vi "Sleep Box.vi"() -> ()   [LabVIEW 2013]
uses:
  <vilib>/DAQmx/write.llb/DAQmx Write (Analog DBL 1Chan 1Samp).vi
  <vilib>/DAQmx/write.llb/DAQmx Write (Digital Bool 1Line 1Point).vi
  <vilib>/DAQmx/miscellaneous.llb/DAQmx Fill In Error Info.vi
panel:
  out "time log 2":refnum<file>
  out "time log":refnum<file>
  out "doQueue2":refnum<queue>
  out "doQueue1":refnum<queue>
  out "camera2":refnum<queue>
  out "camera1":refnum<queue>
  out "integral2":refnum<queue>
  out "integral1":refnum<queue>
  out "centroids2":refnum<queue>
  out "centroids1":refnum<queue>
  out "display2":refnum<queue>
  out "display1":refnum<queue>
  out "threshDisplay2":refnum<queue>
  out "threshDisplay1":refnum<queue>
  in  "roi data cluster 2":T1
  out "ROIs 2":T1={[0, 0, 1280, 960], [{"Contour Type"=0, "ROI Type"=12, [49, 61, 150, 162, 270516]}, {"Contour Type"=0, "ROI Type"=12, [50, 163, 151, 264, 270516]}, {"Contour Type"=0, "ROI Type"=12, [51, 264, 152, 365, 270516]}, {"Contour Type"=0, "ROI Type"=12, [52, 366, 153, 467, 270516]}, {"Contour Type"=0, "ROI Type"=12, [52, 468, 154, 568, 270516]}, {"Contour Type"=0, "ROI Type"=12, [53, 569, 154, 670, 270516]}, {"Contour Type"=0, "ROI Type"=12, [54, 671, 155, 772, 270516]}, {"Contour Type"=0, "ROI Type"=12, [55, 772, 156, 873, 270516]}, {"Contour Type"=0, "ROI Type"=12, [151, 60, 252, 161, 270516]}, {"Contour Type"=0, "ROI Type"=12, [152, 162, 253, 263, 270516]}, {"Contour Type"=0, "ROI Type"=12, [153, 263, 254, 364, 270516]}, {"Contour Type"=0, "ROI Type"=12, [153, 365, 254, 466, 270516]}, {"Contour Type"=0, "ROI Type"=12, [154, 467, 255, 568, 270516]}, {"Contour Type"=0, "ROI Type"=12, [155, 568, 256, 669, 270516]}, {"Contour Type"=0, "ROI Type"=12, [156, 670, 257, 771, 270516]}, {"Contour Type"=0, "ROI Type"=12, [157, 771, 258, 872, 270516]}, {"Contour Type"=0, "ROI Type"=12, [253, 59, 354, 160, 270516]}, {"Contour Type"=0, "ROI Type"=12, [254, 161, 355, 262, 270516]}, {"Contour Type"=0, "ROI Type"=12, [254, 262, 355, 363, 270516]}, {"Contour Type"=0, "ROI Type"=12, [255, 364, 356, 465, 270516]}, {"Contour Type"=0, "ROI Type"=12, [256, 466, 357, 567, 270516]}, {"Contour Type"=0, "ROI Type"=12, [257, 567, 358, 668, 270516]}, {"Contour Type"=0, "ROI Type"=12, [258, 669, 359, 770, 270516]}, {"Contour Type"=0, "ROI Type"=12, [259, 771, 360, 872, 270516]}, {"Contour Type"=0, "ROI Type"=12, [354, 58, 456, 159, 270516]}, {"Contour Type"=0, "ROI Type"=12, [355, 160, 456, 261, 270516]}, {"Contour Type"=0, "ROI Type"=12, [356, 262, 457, 362, 270516]}, {"Contour Type"=0, "ROI Type"=12, [357, 363, 458, 464, 270516]}, {"Contour Type"=0, "ROI Type"=12, [358, 465, 459, 566, 270516]}, {"Contour Type"=0, "ROI Type"=12, [359, 566, 460, 667, 270516]}, {"Contour Type"=0, "ROI Type"=12, [360, 668, 461, 769, 270516]}, {"Contour Type"=0, "ROI Type"=12, [361, 770, 462, 871, 270516]}, {"Contour Type"=0, "ROI Type"=12, [456, 57, 557, 158, 270516]}, {"Contour Type"=0, "ROI Type"=12, [457, 159, 558, 260, 270516]}, {"Contour Type"=0, "ROI Type"=12, [458, 261, 559, 362, 270516]}, {"Contour Type"=0, "ROI Type"=12, [459, 362, 560, 463, 270516]}, {"Contour Type"=0, "ROI Type"=12, [460, 464, 561, 565, 270516]}, {"Contour Type"=0, "ROI Type"=12, [461, 565, 562, 666, 270516]}, {"Contour Type"=0, "ROI Type"=12, [462, 667, 563, 768, 270516]}, {"Contour Type"=0, "ROI Type"=12, [462, 769, 563, 870, 270516]}, {"Contour Type"=0, "ROI Type"=12, [558, 56, 659, 157, 270516]}, {"Contour Type"=0, "ROI Type"=12, [559, 158, 660, 259, 270516]}, {"Contour Type"=0, "ROI Type"=12, [560, 260, 661, 361, 270516]}, {"Contour Type"=0, "ROI Type"=12, [561, 361, 662, 462, 270516]}, {"Contour Type"=0, "ROI Type"=12, [562, 463, 663, 564, 270516]}, {"Contour Type"=0, "ROI Type"=12, [563, 565, 664, 666, 270516]}, {"Contour Type"=0, "ROI Type"=12, [563, 666, 664, 767, 270516]}, {"Contour Type"=0, "ROI Type"=12, [564, 768, 665, 869, 270516]}, {"Contour Type"=0, "ROI Type"=12, [660, 56, 761, 156, 270516]}, {"Contour Type"=0, "ROI Type"=12, [661, 157, 762, 258, 270516]}, {"Contour Type"=0, "ROI Type"=12, [662, 259, 763, 360, 270516]}, {"Contour Type"=0, "ROI Type"=12, [663, 360, 764, 461, 270516]}, {"Contour Type"=0, "ROI Type"=12, [664, 462, 764, 563, 270516]}, {"Contour Type"=0, "ROI Type"=12, [664, 564, 765, 665, 270516]}, {"Contour Type"=0, "ROI Type"=12, [665, 665, 766, 766, 270516]}, {"Contour Type"=0, "ROI Type"=12, [666, 767, 767, 868, 270516]}, {"Contour Type"=0, "ROI Type"=12, [762, 55, 863, 156, 270516]}, {"Contour Type"=0, "ROI Type"=12, [763, 156, 864, 257, 270516]}, {"Contour Type"=0, "ROI Type"=12, [764, 258, 865, 359, 270516]}, {"Contour Type"=0, "ROI Type"=12, [764, 359, 865, 460, 270516]}, {"Contour Type"=0, "ROI Type"=12, [765, 461, 866, 562, 270516]}, {"Contour Type"=0, "ROI Type"=12, [766, 563, 867, 664, 270516]}, {"Contour Type"=0, "ROI Type"=12, [767, 664, 868, 765, 270516]}, {"Contour Type"=0, "ROI Type"=12, [768, 766, 869, 867, 270516]}, {"Contour Type"=0, "ROI Type"=12, [864, 54, 965, 155, 270516]}, {"Contour Type"=0, "ROI Type"=12, [865, 155, 966, 256, 270516]}, {"Contour Type"=0, "ROI Type"=12, [865, 257, 966, 358, 270516]}, {"Contour Type"=0, "ROI Type"=12, [866, 359, 967, 460, 270516]}, {"Contour Type"=0, "ROI Type"=12, [867, 460, 968, 561, 270516]}, {"Contour Type"=0, "ROI Type"=12, [868, 562, 969, 663, 270516]}, {"Contour Type"=0, "ROI Type"=12, [869, 663, 970, 764, 270516]}, {"Contour Type"=0, "ROI Type"=12, [870, 765, 971, 866, 270516]}, {"Contour Type"=0, "ROI Type"=12, [966, 53, 1066, 154, 270516]}, {"Contour Type"=0, "ROI Type"=12, [966, 154, 1067, 255, 270516]}, {"Contour Type"=0, "ROI Type"=12, [967, 256, 1068, 357, 270516]}, {"Contour Type"=0, "ROI Type"=12, [968, 358, 1069, 459, 270516]}, {"Contour Type"=0, "ROI Type"=12, [969, 459, 1070, 560, 270516]}, {"Contour Type"=0, "ROI Type"=12, [970, 561, 1071, 662, 270516]}, {"Contour Type"=0, "ROI Type"=12, [971, 662, 1072, 764, 270516]}, {"Contour Type"=0, "ROI Type"=12, [972, 764, 1073, 865, 270516]}, {"Contour Type"=0, "ROI Type"=12, [1067, 52, 1168, 153, 270516]}, {"Contour Type"=0, "ROI Type"=12, [1068, 153, 1169, 254, 270516]}, {"Contour Type"=0, "ROI Type"=12, [1069, 255, 1170, 356, 270516]}, {"Contour Type"=0, "ROI Type"=12, [1070, 357, 1171, 458, 270516]}, {"Contour Type"=0, "ROI Type"=12, [1071, 458, 1172, 559, 270516]}, {"Contour Type"=0, "ROI Type"=12, [1072, 560, 1173, 661, 270516]}, {"Contour Type"=0, "ROI Type"=12, [1073, 662, 1174, 763, 270516]}, {"Contour Type"=0, "ROI Type"=12, [1073, 763, 1174, 864, 270516]}, {"Contour Type"=0, "ROI Type"=12, [1169, 51, 1270, 152, 270516]}, {"Contour Type"=0, "ROI Type"=12, [1170, 153, 1271, 254, 270516]}, {"Contour Type"=0, "ROI Type"=12, [1171, 254, 1272, 355, 270516]}, {"Contour Type"=0, "ROI Type"=12, [1172, 356, 1273, 457, 270516]}, {"Contour Type"=0, "ROI Type"=12, [1173, 457, 1274, 558, 270516]}, {"Contour Type"=0, "ROI Type"=12, [1174, 559, 1275, 660, 270516]}, {"Contour Type"=0, "ROI Type"=12, [1174, 661, 1275, 762, 270516]}, {"Contour Type"=0, "ROI Type"=12, [1175, 762, 1276, 863, 270516]}]}
  out "centroid log 2":refnum<file>
  out "motion log 2":refnum<file>
  in  "Tab Control":enum32{"Main View", "Files to load/save"}(tab)=enum."Files to load/save"
  out "Image":T2(plugin-control)
  in  "Camera":bool=TRUE
  in  "Ring":u16(ring) items=["Raw", "Diff Threshold", "Integrated Motion"]
  in  "stop":bool
  out "Buffers":i32(slide) scale=0.0..100.0
  out "Intensity Graph":u32[][](graph)
  out "frame#1":i32
  out "frame#2":i32
  in  "ROI Refernce Image 2":path=path "C:/Users/SleepBox/Desktop/072516_Box4.bmp"
  in  "ROI Refernce Image 1":path=path "C:/Users/SleepBox/Desktop/072516_Box3.bmp"
  in  "Load Experimental Parameters 2":path=path "C:/Users/SleepBox/Desktop/072516_TapsFlashes_Box4_Complete.csv"
  in  "Load ROI Data 2":path=path "C:/Users/SleepBox/Desktop/072516_Box4_ROI"
  in  "Log File Base Name 2":path=path "C:/Users/SleepBox/Desktop/testlog"
  in  "Load Experimental Parameters":path=path "C:/Users/SleepBox/Desktop/072516_TapsFlashes_Box3_Complete.csv"
  in  "Load ROI Data":path=path "C:/Users/SleepBox/Desktop/072516_Box3_ROI"
  in  "Log File Base Name":path=path "C:/Users/SleepBox/Desktop/testlog"
  in  "diff threshold":dbl=3.0
  out "event log":refnum<file>
  out "event log 2":refnum<file>
  out "motion log":refnum<file>
  out "centroid log":refnum<file>
  out "ROIs":T1={[0, 0, 1280, 960], [{"Contour Type"=0, "ROI Type"=12, [49, 61, 150, 162, 270516]}, {"Contour Type"=0, "ROI Type"=12, [50, 163, 151, 264, 270516]}, {"Contour Type"=0, "ROI Type"=12, [51, 264, 152, 365, 270516]}, {"Contour Type"=0, "ROI Type"=12, [52, 366, 153, 467, 270516]}, {"Contour Type"=0, "ROI Type"=12, [52, 468, 154, 568, 270516]}, {"Contour Type"=0, "ROI Type"=12, [53, 569, 154, 670, 270516]}, {"Contour Type"=0, "ROI Type"=12, [54, 671, 155, 772, 270516]}, {"Contour Type"=0, "ROI Type"=12, [55, 772, 156, 873, 270516]}, {"Contour Type"=0, "ROI Type"=12, [151, 60, 252, 161, 270516]}, {"Contour Type"=0, "ROI Type"=12, [152, 162, 253, 263, 270516]}, {"Contour Type"=0, "ROI Type"=12, [153, 263, 254, 364, 270516]}, {"Contour Type"=0, "ROI Type"=12, [153, 365, 254, 466, 270516]}, {"Contour Type"=0, "ROI Type"=12, [154, 467, 255, 568, 270516]}, {"Contour Type"=0, "ROI Type"=12, [155, 568, 256, 669, 270516]}, {"Contour Type"=0, "ROI Type"=12, [156, 670, 257, 771, 270516]}, {"Contour Type"=0, "ROI Type"=12, [157, 771, 258, 872, 270516]}, {"Contour Type"=0, "ROI Type"=12, [253, 59, 354, 160, 270516]}, {"Contour Type"=0, "ROI Type"=12, [254, 161, 355, 262, 270516]}, {"Contour Type"=0, "ROI Type"=12, [254, 262, 355, 363, 270516]}, {"Contour Type"=0, "ROI Type"=12, [255, 364, 356, 465, 270516]}, {"Contour Type"=0, "ROI Type"=12, [256, 466, 357, 567, 270516]}, {"Contour Type"=0, "ROI Type"=12, [257, 567, 358, 668, 270516]}, {"Contour Type"=0, "ROI Type"=12, [258, 669, 359, 770, 270516]}, {"Contour Type"=0, "ROI Type"=12, [259, 771, 360, 872, 270516]}, {"Contour Type"=0, "ROI Type"=12, [354, 58, 456, 159, 270516]}, {"Contour Type"=0, "ROI Type"=12, [355, 160, 456, 261, 270516]}, {"Contour Type"=0, "ROI Type"=12, [356, 262, 457, 362, 270516]}, {"Contour Type"=0, "ROI Type"=12, [357, 363, 458, 464, 270516]}, {"Contour Type"=0, "ROI Type"=12, [358, 465, 459, 566, 270516]}, {"Contour Type"=0, "ROI Type"=12, [359, 566, 460, 667, 270516]}, {"Contour Type"=0, "ROI Type"=12, [360, 668, 461, 769, 270516]}, {"Contour Type"=0, "ROI Type"=12, [361, 770, 462, 871, 270516]}, {"Contour Type"=0, "ROI Type"=12, [456, 57, 557, 158, 270516]}, {"Contour Type"=0, "ROI Type"=12, [457, 159, 558, 260, 270516]}, {"Contour Type"=0, "ROI Type"=12, [458, 261, 559, 362, 270516]}, {"Contour Type"=0, "ROI Type"=12, [459, 362, 560, 463, 270516]}, {"Contour Type"=0, "ROI Type"=12, [460, 464, 561, 565, 270516]}, {"Contour Type"=0, "ROI Type"=12, [461, 565, 562, 666, 270516]}, {"Contour Type"=0, "ROI Type"=12, [462, 667, 563, 768, 270516]}, {"Contour Type"=0, "ROI Type"=12, [462, 769, 563, 870, 270516]}, {"Contour Type"=0, "ROI Type"=12, [558, 56, 659, 157, 270516]}, {"Contour Type"=0, "ROI Type"=12, [559, 158, 660, 259, 270516]}, {"Contour Type"=0, "ROI Type"=12, [560, 260, 661, 361, 270516]}, {"Contour Type"=0, "ROI Type"=12, [561, 361, 662, 462, 270516]}, {"Contour Type"=0, "ROI Type"=12, [562, 463, 663, 564, 270516]}, {"Contour Type"=0, "ROI Type"=12, [563, 565, 664, 666, 270516]}, {"Contour Type"=0, "ROI Type"=12, [563, 666, 664, 767, 270516]}, {"Contour Type"=0, "ROI Type"=12, [564, 768, 665, 869, 270516]}, {"Contour Type"=0, "ROI Type"=12, [660, 56, 761, 156, 270516]}, {"Contour Type"=0, "ROI Type"=12, [661, 157, 762, 258, 270516]}, {"Contour Type"=0, "ROI Type"=12, [662, 259, 763, 360, 270516]}, {"Contour Type"=0, "ROI Type"=12, [663, 360, 764, 461, 270516]}, {"Contour Type"=0, "ROI Type"=12, [664, 462, 764, 563, 270516]}, {"Contour Type"=0, "ROI Type"=12, [664, 564, 765, 665, 270516]}, {"Contour Type"=0, "ROI Type"=12, [665, 665, 766, 766, 270516]}, {"Contour Type"=0, "ROI Type"=12, [666, 767, 767, 868, 270516]}, {"Contour Type"=0, "ROI Type"=12, [762, 55, 863, 156, 270516]}, {"Contour Type"=0, "ROI Type"=12, [763, 156, 864, 257, 270516]}, {"Contour Type"=0, "ROI Type"=12, [764, 258, 865, 359, 270516]}, {"Contour Type"=0, "ROI Type"=12, [764, 359, 865, 460, 270516]}, {"Contour Type"=0, "ROI Type"=12, [765, 461, 866, 562, 270516]}, {"Contour Type"=0, "ROI Type"=12, [766, 563, 867, 664, 270516]}, {"Contour Type"=0, "ROI Type"=12, [767, 664, 868, 765, 270516]}, {"Contour Type"=0, "ROI Type"=12, [768, 766, 869, 867, 270516]}, {"Contour Type"=0, "ROI Type"=12, [864, 54, 965, 155, 270516]}, {"Contour Type"=0, "ROI Type"=12, [865, 155, 966, 256, 270516]}, {"Contour Type"=0, "ROI Type"=12, [865, 257, 966, 358, 270516]}, {"Contour Type"=0, "ROI Type"=12, [866, 359, 967, 460, 270516]}, {"Contour Type"=0, "ROI Type"=12, [867, 460, 968, 561, 270516]}, {"Contour Type"=0, "ROI Type"=12, [868, 562, 969, 663, 270516]}, {"Contour Type"=0, "ROI Type"=12, [869, 663, 970, 764, 270516]}, {"Contour Type"=0, "ROI Type"=12, [870, 765, 971, 866, 270516]}, {"Contour Type"=0, "ROI Type"=12, [966, 53, 1066, 154, 270516]}, {"Contour Type"=0, "ROI Type"=12, [966, 154, 1067, 255, 270516]}, {"Contour Type"=0, "ROI Type"=12, [967, 256, 1068, 357, 270516]}, {"Contour Type"=0, "ROI Type"=12, [968, 358, 1069, 459, 270516]}, {"Contour Type"=0, "ROI Type"=12, [969, 459, 1070, 560, 270516]}, {"Contour Type"=0, "ROI Type"=12, [970, 561, 1071, 662, 270516]}, {"Contour Type"=0, "ROI Type"=12, [971, 662, 1072, 764, 270516]}, {"Contour Type"=0, "ROI Type"=12, [972, 764, 1073, 865, 270516]}, {"Contour Type"=0, "ROI Type"=12, [1067, 52, 1168, 153, 270516]}, {"Contour Type"=0, "ROI Type"=12, [1068, 153, 1169, 254, 270516]}, {"Contour Type"=0, "ROI Type"=12, [1069, 255, 1170, 356, 270516]}, {"Contour Type"=0, "ROI Type"=12, [1070, 357, 1171, 458, 270516]}, {"Contour Type"=0, "ROI Type"=12, [1071, 458, 1172, 559, 270516]}, {"Contour Type"=0, "ROI Type"=12, [1072, 560, 1173, 661, 270516]}, {"Contour Type"=0, "ROI Type"=12, [1073, 662, 1174, 763, 270516]}, {"Contour Type"=0, "ROI Type"=12, [1073, 763, 1174, 864, 270516]}, {"Contour Type"=0, "ROI Type"=12, [1169, 51, 1270, 152, 270516]}, {"Contour Type"=0, "ROI Type"=12, [1170, 153, 1271, 254, 270516]}, {"Contour Type"=0, "ROI Type"=12, [1171, 254, 1272, 355, 270516]}, {"Contour Type"=0, "ROI Type"=12, [1172, 356, 1273, 457, 270516]}, {"Contour Type"=0, "ROI Type"=12, [1173, 457, 1274, 558, 270516]}, {"Contour Type"=0, "ROI Type"=12, [1174, 559, 1275, 660, 270516]}, {"Contour Type"=0, "ROI Type"=12, [1174, 661, 1275, 762, 270516]}, {"Contour Type"=0, "ROI Type"=12, [1175, 762, 1276, 863, 270516]}]}
  in  "roi data cluster":T1
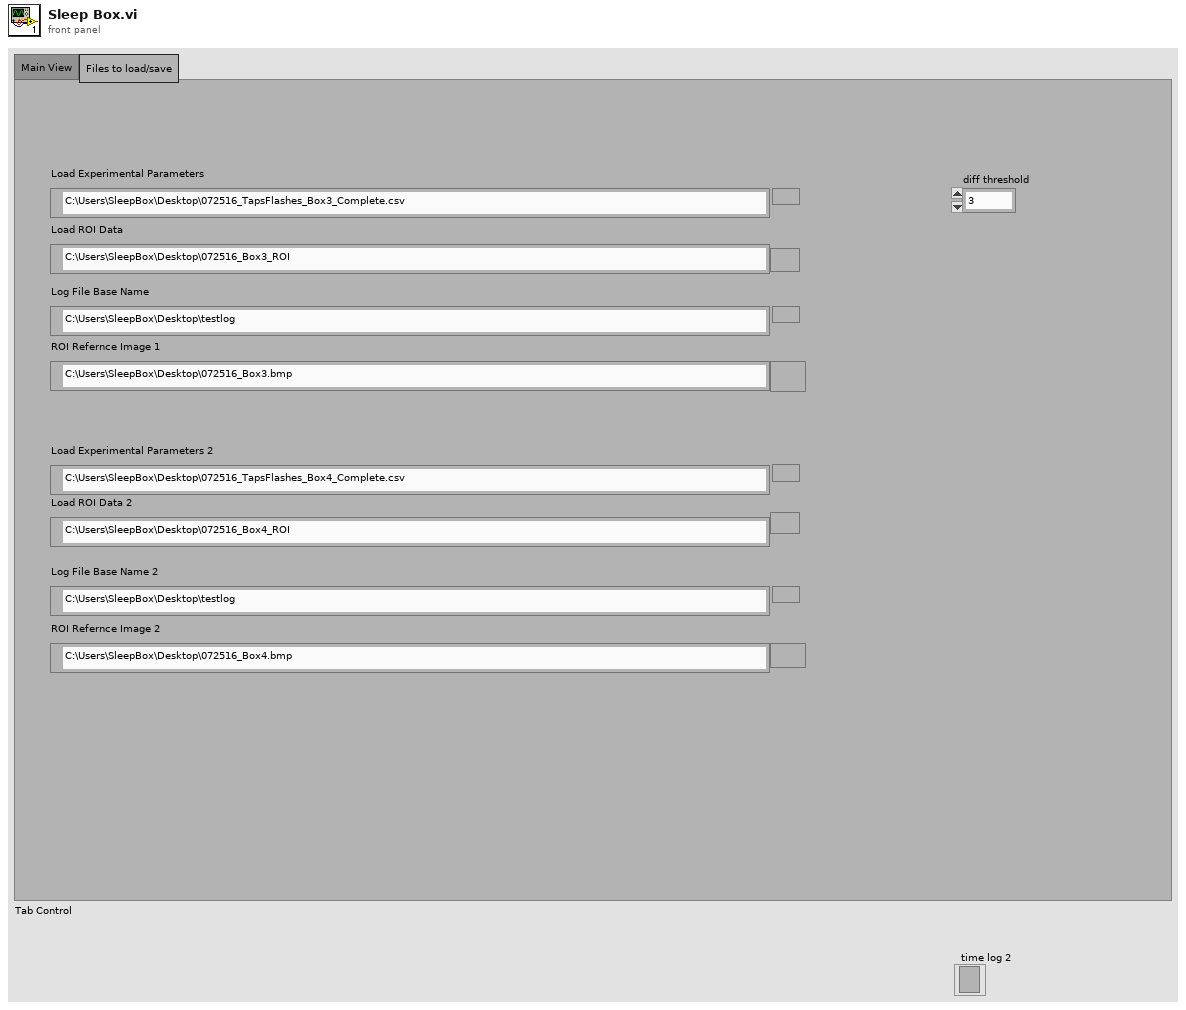
[diagram p1: front panel]
types:
  T1 = cluster{i32[], cluster{"Contour Type":u32, "ROI Type":u32, i32[]}[]}
  T2 = typedef "IMAQ Image.ctl" = refnum<image>
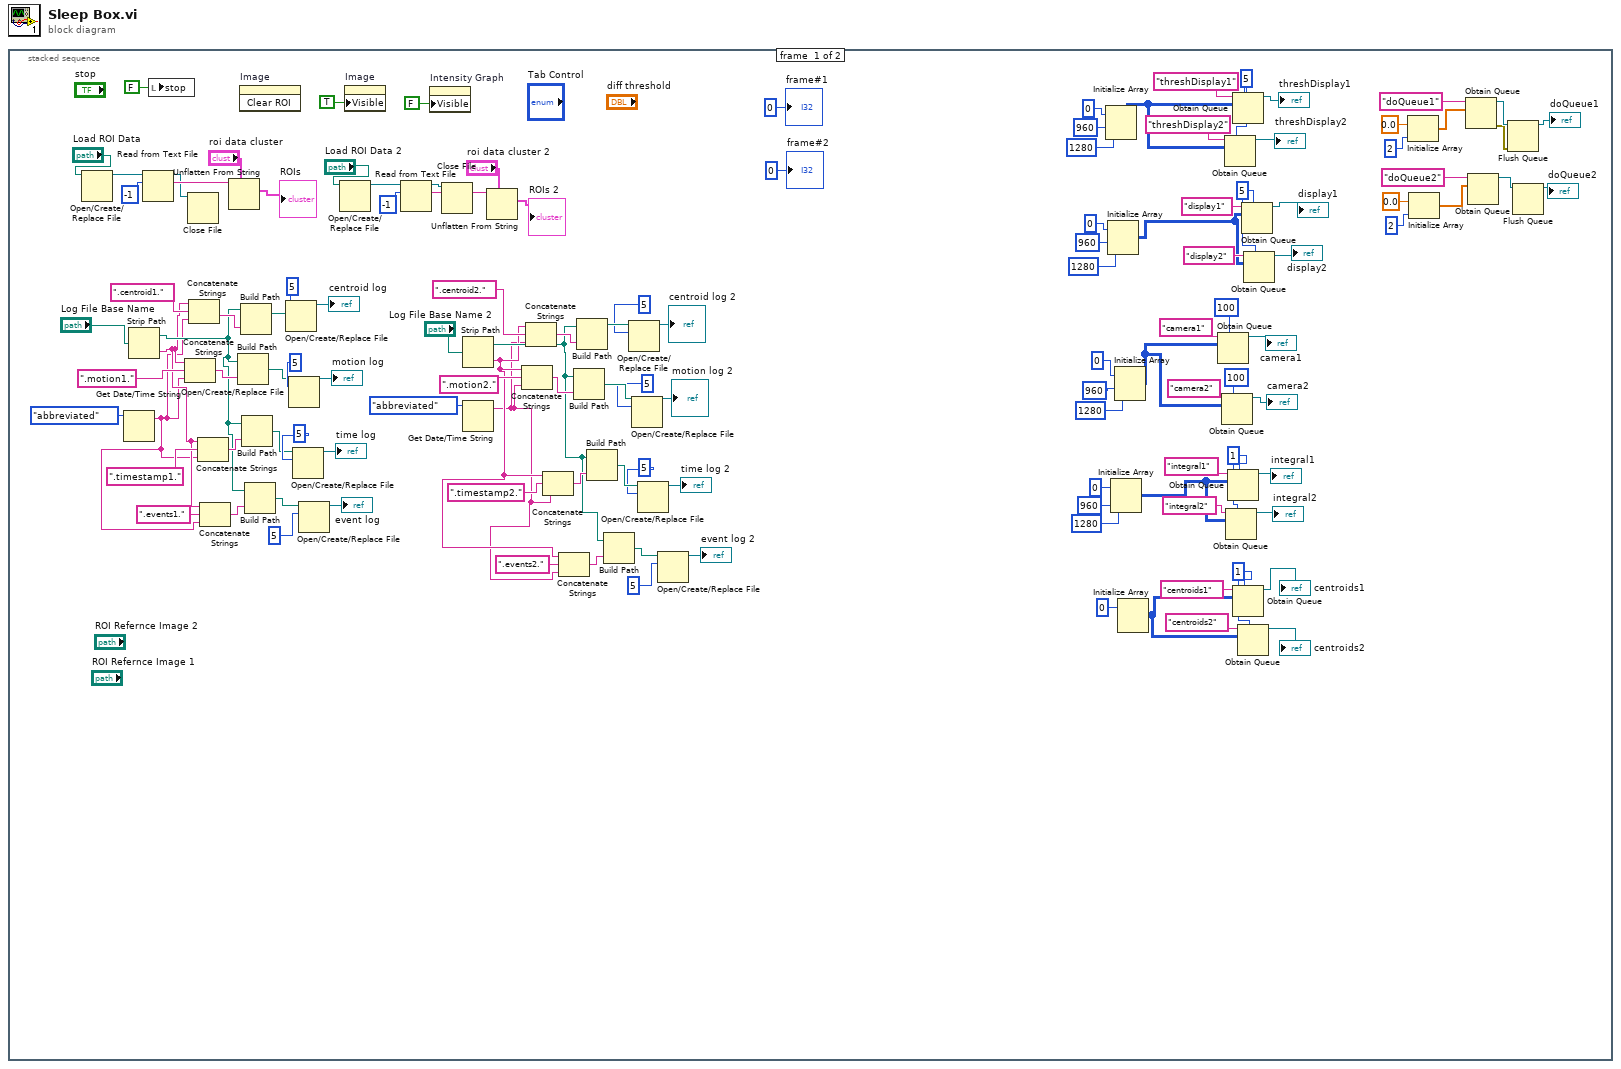
[diagram p0: block diagram]
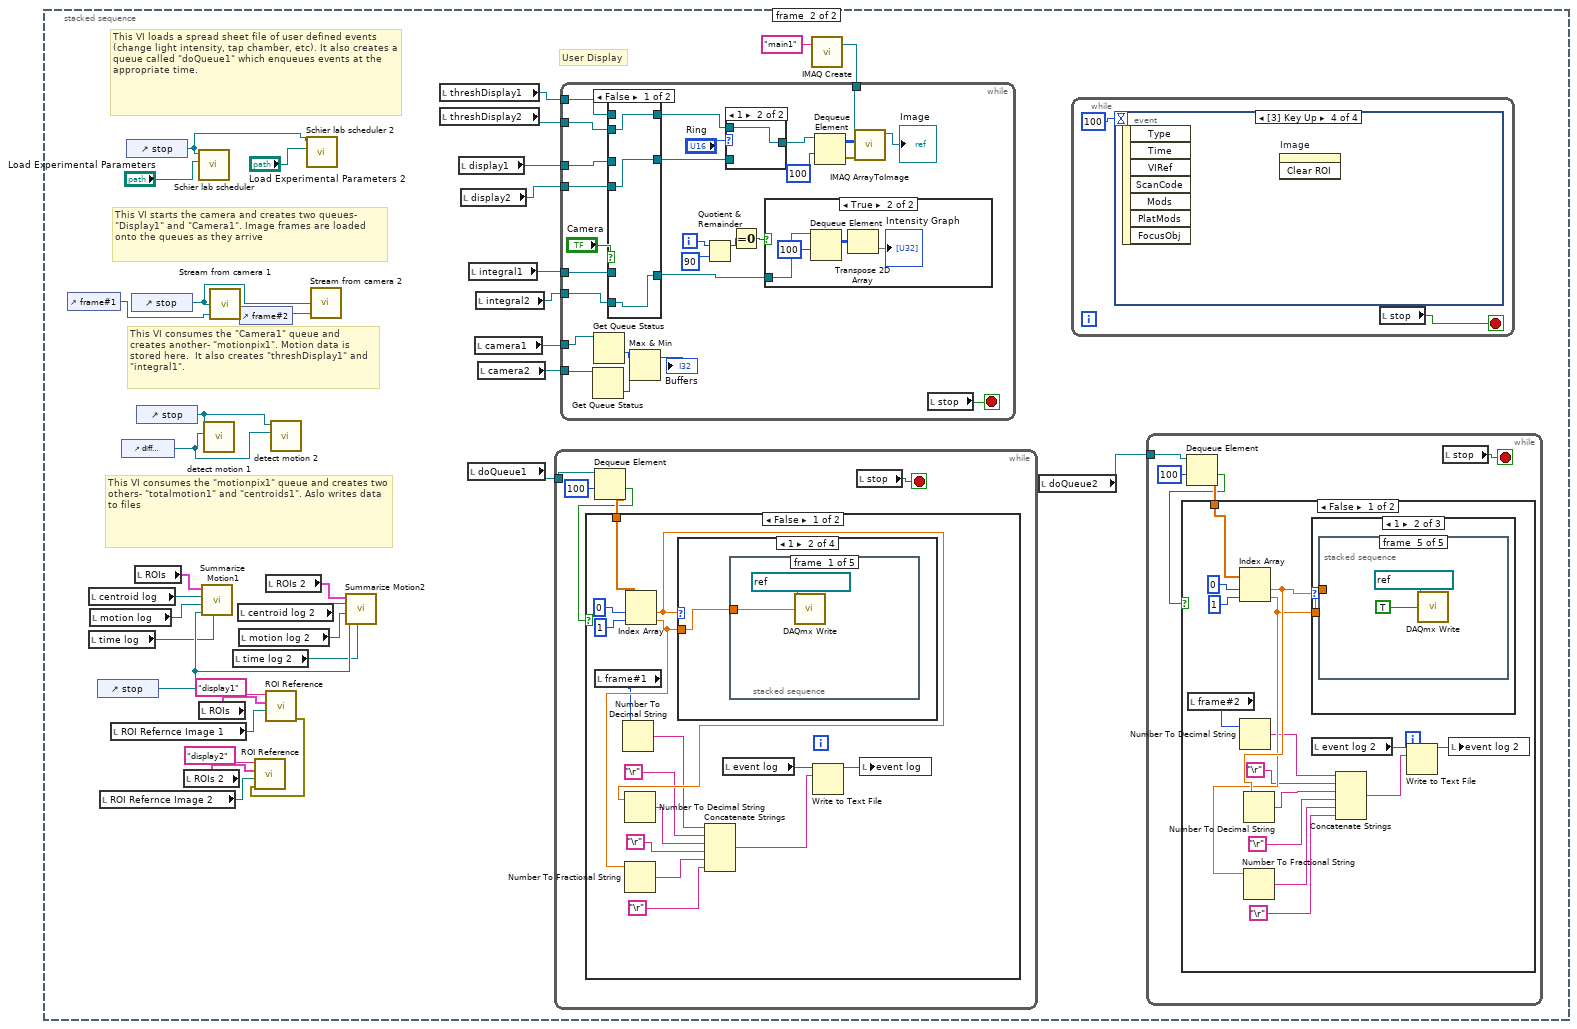
[diagram p2: hidden frame]
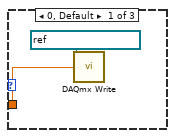
[diagram p3: hidden frame]
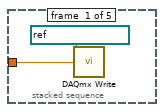
[diagram p4: hidden frame]
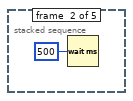
[diagram p5: hidden frame]
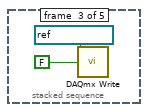
[diagram p6: hidden frame]
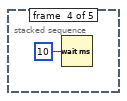
[diagram p7: hidden frame]
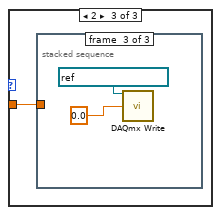
[diagram p8: hidden frame]
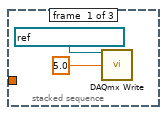
[diagram p9: hidden frame]
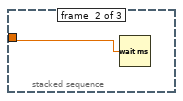
[diagram p10: hidden frame]
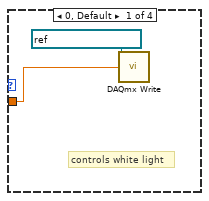
[diagram p12: hidden frame]
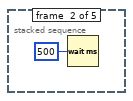
[diagram p13: hidden frame]
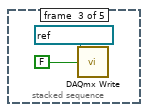
[diagram p14: hidden frame]
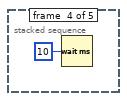
[diagram p15: hidden frame]
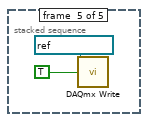
[diagram p16: hidden frame]
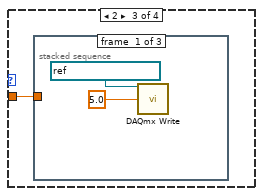
[diagram p17: hidden frame]
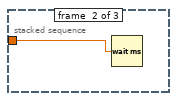
[diagram p18: hidden frame]
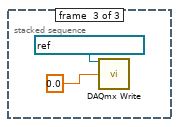
[diagram p19: hidden frame]
diagram:
  n1 = stacked-sequence {
    frame #0 {
      w46 = 1 ("max queue size (-1, unlimited)")
      w61 = 1 ("max queue size (-1, unlimited)")
      w70 = 5 ("max queue size (-1, unlimited)")
      w77 = 5 ("max queue size (-1, unlimited)")
      n2 = Open/Create/Replace File(file path (use dialog)="Load ROI Data") -> (refnum out=w121:refnum<file>)  [unwired: 5 in, 2 out]
      n3 = Get Date/Time String(date format (0)=enum16{"short", "long", "abbreviated"}."abbreviated") -> (date string=w18:string)  [unwired: 2 in, 1 out]
      n4 = Strip Path(path="Log File Base Name") -> (stripped path=w21:path, name=w20:string)
      n5 = Read from Text File(file (use dialog)=w121, count=-1) -> (refnum out=w123:refnum<file>, text=w124:string)  [unwired: 2 in, 2 out]
      n6 = local write "stop"(FALSE ("stop")) -> ()
      n7 = Concatenate Strings(w20, ".motion1.", w18) -> (w112:string)
      n8 = Close File(refnum=w123) -> ()  [unwired: 1 in, 2 out]
      n9 = Concatenate Strings(w20, ".centroid1.", w18) -> (w113:string)
      n10 = Concatenate Strings(w20, ".timestamp1." ("string"), w18) -> (w32:string)
      n11 = Concatenate Strings(w20, ".events1." ("string"), w18) -> (w23:string)
      n12 = Unflatten From String(type="roi data cluster", binary string=w124) -> (value=→"ROIs":T1)  [unwired: 3 in, 2 out]
      n13 = Build Path(base path=w21, name or relative path=w112) -> (appended path=w108:path)
      n14 = invoke on="Image" class="ImageControl" method="Clear ROI"() -> ()  [unwired: 3 in, 3 out]
      n15 = Build Path(base path=w21, name or relative path=w113) -> (appended path=w111:path)
      n16 = Build Path(base path=w21, name or relative path=w32) -> (appended path=w30:path)
      n17 = Build Path(base path=w21, name or relative path=w23) -> (appended path=w22:path)
      n18 = Open/Create/Replace File(file path (use dialog)=w111, operation (0:open)=5 ("count")) -> (refnum out=→"centroid log":refnum<file>)  [unwired: 4 in, 2 out]
      n19 = Open/Create/Replace File(file path (use dialog)=w108, operation (0:open)=5 ("count")) -> (refnum out=→"motion log":refnum<file>)  [unwired: 4 in, 2 out]
      n20 = Open/Create/Replace File(file path (use dialog)=w30, operation (0:open)=5 ("count")) -> (refnum out=→"time log":refnum<file>)  [unwired: 4 in, 2 out]
      n21 = Open/Create/Replace File(file path (use dialog)=w22, operation (0:open)=5 ("count")) -> (refnum out=→"event log":refnum<file>)  [unwired: 4 in, 2 out]
      n22 = Open/Create/Replace File(file path (use dialog)="Load ROI Data 2") -> (refnum out=w94:refnum<file>)  [unwired: 5 in, 2 out]
      n23 = property on="Image" class="ImageControl"("Visible"=TRUE) -> ()  [unwired: 2 in, 2 out]
      n24 = Read from Text File(file (use dialog)=w94, count=-1) -> (refnum out=w92:refnum<file>, text=w91:string)  [unwired: 2 in, 2 out]
      n25 = property on="Intensity Graph" class="IntGraph (strict)"("Visible"=FALSE) -> ()  [unwired: 2 in, 2 out]
      n26 = Close File(refnum=w92) -> ()  [unwired: 1 in, 2 out]
      n27 = Strip Path(path="Log File Base Name 2") -> (stripped path=w12:path, name=w11:string)
      n28 = Get Date/Time String(date format (0)=enum16{"short", "long", "abbreviated"}."abbreviated") -> (date string=w10:string)  [unwired: 2 in, 1 out]
      n29 = Unflatten From String(type="roi data cluster 2", binary string=w91) -> (value=→"ROIs 2":T1)  [unwired: 3 in, 2 out]
      n30 = Concatenate Strings(w11, ".motion2.", w10) -> (w103:string)
      n31 = Concatenate Strings(w11, ".centroid2.", w10) -> (w102:string)
      n32 = Concatenate Strings(w11, ".timestamp2." ("string"), w10) -> (w25:string)
      n33 = Concatenate Strings(w11, ".events2." ("string"), w10) -> (w13:string)
      n34 = Build Path(base path=w12, name or relative path=w103) -> (appended path=w107:path)
      n35 = Build Path(base path=w12, name or relative path=w102) -> (appended path=w104:path)
      n36 = Build Path(base path=w12, name or relative path=w25) -> (appended path=w27:path)
      n37 = Build Path(base path=w12, name or relative path=w13) -> (appended path=w14:path)
      n38 = Open/Create/Replace File(file path (use dialog)=w104, operation (0:open)=5 ("count")) -> (refnum out=→"centroid log 2":refnum<file>)  [unwired: 4 in, 2 out]
      n39 = Open/Create/Replace File(file path (use dialog)=w107, operation (0:open)=5 ("count")) -> (refnum out=→"motion log 2":refnum<file>)  [unwired: 4 in, 2 out]
      n40 = Open/Create/Replace File(file path (use dialog)=w27, operation (0:open)=5 ("count")) -> (refnum out=→"time log 2":refnum<file>)  [unwired: 4 in, 2 out]
      n41 = Open/Create/Replace File(file path (use dialog)=w14, operation (0:open)=5 ("count")) -> (refnum out=→"event log 2":refnum<file>)  [unwired: 4 in, 2 out]
      n42 = Initialize Array(u8 0 ("element"), 960 ("dimension size"), 1280 ("dimension size")) -> (w79:u8[][])
      n43 = Initialize Array(u8 0 ("element"), 960 ("dimension size"), 1280 ("dimension size")) -> (w69:u8[][])
      n44 = Initialize Array(u32 0 ("element"), 960 ("dimension size"), 1280 ("dimension size")) -> (w62:u32[][])
      n45 = Initialize Array(i16 0 ("element"), 960 ("dimension size"), 1280 ("dimension size")) -> (w42:i16[][])
      n46 = Initialize Array(u16 0 ("element")) -> (w45:u16[][])  [unwired: 2 in]
      n47 = Obtain Queue(max queue size (-1, unlimited)=100, name (unnamed)="camera1", element data type=w42) -> (queue out=→"camera1":refnum<queue>)  [unwired: 2 in, 2 out]
      n48 = Obtain Queue(max queue size (-1, unlimited)=100, name (unnamed)="camera2", element data type=w42) -> (queue out=→"camera2":refnum<queue>)  [unwired: 2 in, 2 out]
      n49 = Obtain Queue(max queue size (-1, unlimited)=w77, name (unnamed)="threshDisplay2", element data type=w79) -> (queue out=→"threshDisplay2":refnum<queue>)  [unwired: 2 in, 2 out]
      n50 = Obtain Queue(max queue size (-1, unlimited)=w61, name (unnamed)="integral2", element data type=w62) -> (queue out=→"integral2":refnum<queue>)  [unwired: 2 in, 2 out]
      n51 = Obtain Queue(max queue size (-1, unlimited)=w61, name (unnamed)="integral1", element data type=w62) -> (queue out=→"integral1":refnum<queue>)  [unwired: 2 in, 2 out]
      n52 = Obtain Queue(max queue size (-1, unlimited)=w77, name (unnamed)="threshDisplay1", element data type=w79) -> (queue out=→"threshDisplay1":refnum<queue>)  [unwired: 2 in, 2 out]
      n53 = Obtain Queue(max queue size (-1, unlimited)=w46, name (unnamed)="centroids1", element data type=w45) -> (queue out=→"centroids1":refnum<queue>)  [unwired: 2 in, 2 out]
      n54 = Obtain Queue(max queue size (-1, unlimited)=w46, name (unnamed)="centroids2", element data type=w45) -> (queue out=→"centroids2":refnum<queue>)  [unwired: 2 in, 2 out]
      n55 = Obtain Queue(max queue size (-1, unlimited)=w70, name (unnamed)="display1", element data type=w69) -> (queue out=→"display1":refnum<queue>)  [unwired: 2 in, 2 out]
      n56 = Obtain Queue(max queue size (-1, unlimited)=w70, name (unnamed)="display2", element data type=w69) -> (queue out=→"display2":refnum<queue>)  [unwired: 2 in, 2 out]
      n57 = Initialize Array(0.0 ("element"), 2 ("dimension size")) -> (w34:dbl[])
      n58 = Initialize Array(0.0 ("element"), 2 ("dimension size")) -> (w38:dbl[])
      n59 = Obtain Queue(name (unnamed)="doQueue1", element data type=w34) -> (queue out=w3:refnum<queue>, error out=w2:errorcluster)  [unwired: 3 in, 1 out]
      n60 = Obtain Queue(name (unnamed)="doQueue2", element data type=w38) -> (queue out=w5:refnum<queue>)  [unwired: 3 in, 2 out]
      n61 = Flush Queue(queue=w3, error in (no error)=w2) -> (queue out=→"doQueue1":refnum<queue>)  [unwired: 2 out]
      n62 = Flush Queue(queue=w5) -> (queue out=→"doQueue2":refnum<queue>)  [unwired: 1 in, 2 out]
      "frame#1" <- 0 ("frame#1")
      "frame#2" <- 0 ("frame#2")
    }
    frame #1 {
      # "User Display"
      # "This VI consumes the \"motionpix1\" queue and creates two others- \"totalmotion1\" and \"centroids1\". Aslo writes data to files"
      # "This VI consumes the \"Camera1\" queue and creates another- \"motionpix1\". Motion data is stored here.  It also creates \"threshDisplay1\" and \"integral1\"."
      # "This VI starts the camera and creates two queues- \"Display1\" and \"Camera1\". Image frames are loaded onto the queues as they arrive"
      # "This VI loads a spread sheet file of user defined events (change light intensity, tap chamber, etc). It also creates a queue called \"doQueue1\" which enqueues events at the appropriate time."
      n63 = control-ref of="frame#1"() -> (w128:refnum<vi>)
      n64 = local read "centroid log"() -> (w153:refnum<file>)
      n65 = local read "time log"() -> (w133:refnum<file>)
      n66 = local read "motion log"() -> (w152:refnum<file>)
      n67 = control-ref of="stop"() -> (w148:refnum<vi>)
      n68 = local read "ROI Refernce Image 2"() -> (w129:path)
      n69 = local read "ROI Refernce Image 1"() -> (w137:path)
      n70 = control-ref of="diff threshold"() -> (w157:refnum<vi>)
      n71 = control-ref of="stop"() -> (w155:refnum<vi>)
      n72 = control-ref of="stop"() -> (w159:refnum<vi>)
      n73 = local read "ROIs"() -> (w154:T1)
      n74 = control-ref of="stop"() -> (w158:refnum<vi>)
      n75 = local read "ROIs 2"() -> (w130:T1)
      n76 = call "Schier lab scheduler.vi"("Load Experimental Parameters"="Load Experimental Parameters", "External Stop"=w155) -> ()  [unwired: 9 in, 1 out]
      n77 = local read "ROIs"() -> (w136:T1)
      n78 = call "Summarize Motion1.vi"("time log"=w133, "external stop"=w148, "motion log"=w152, "centroid log"=w153, "roi data cluster"=w154) -> ()  [unwired: 7 in]
      n79 = call "detect motion 1.vi"("thresh 1"=w157, "external stop"=w158) -> ()  [unwired: 10 in]
      n80 = call "Stream from camera 1.vi"("frame#"=w128, "External Stop"=w159) -> ()  [unwired: 2 in]
      n81 = local read "time log 2"() -> (w132:refnum<file>)
      n82 = local read "centroid log 2"() -> (w150:refnum<file>)
      n83 = local read "motion log 2"() -> (w151:refnum<file>)
      n84 = control-ref of="frame#2"() -> (w127:refnum<vi>)
      n85 = local read "ROIs 2"() -> (w149:T1)
      n86 = call "ROI Reference.vi"("Path"=w137, "ROIs"=w136, "queue name"="display1") -> ("error out"=w134:errorcluster)  [unwired: 8 in]
      n87 = call "ROI Reference.vi"("error in (no error)"=w134, "Path"=w129, "ROIs"=w130, "queue name"="display2") -> ()  [unwired: 7 in, 1 out]
      n88 = call "detect motion 2.vi"("thresh 1"=w157, "external stop"=w158) -> ()  [unwired: 10 in]
      n89 = call "Schier lab scheduler 2.vi"("Load Experimental Parameters"="Load Experimental Parameters 2", "External Stop"=w155) -> ()  [unwired: 9 in, 1 out]
      n90 = call "Stream from camera 2.vi"("frame#"=w127, "External Stop"=w159) -> ()  [unwired: 2 in]
      n91 = call "Summarize Motion2.vi"("time log"=w132, "external stop"=w148, "motion log"=w151, "centroid log"=w150, "roi data cluster"=w149) -> ()  [unwired: 7 in]
      n92 = local read "threshDisplay1"() -> (w147:refnum<queue>)
      n93 = local read "threshDisplay2"() -> (w146:refnum<queue>)
      n94 = local read "display1"() -> (w145:refnum<queue>)
      n95 = local read "display2"() -> (w144:refnum<queue>)
      n96 = local read "doQueue1"() -> (w139:refnum<queue>)
      n97 = local read "integral1"() -> (w143:refnum<queue>)
      n98 = local read "camera1"() -> (w141:refnum<queue>)
      n99 = local read "integral2"() -> (w142:refnum<queue>)
      n100 = local read "camera2"() -> (w140:refnum<queue>)
      n101 = while {
        tunnel: w139 -> [w203]
        stop <- w204 stop-if-true
        n102 = Dequeue Element(queue=w203, timeout in ms (-1)=100) -> (element=w201:dbl[], timed out?=w200:bool)  [unwired: 1 in, 2 out]
        n103 = case shown="False" w200 {
          tunnel: w201 -> [w219 _]
          frame False {
            n104 = local read "frame#1"() -> (w211:i32)
            n105 = Number To Decimal String(number=w211) -> (decimal integer string=w210:string)  [unwired: 1 in]
            n106 = Index Array(array=w219, index #1=0 ("index"), index #2=1 ("index")) -> (element #1=w213:dbl, element #2=w214:dbl)
            n107 = Number To Decimal String(number=w213) -> (decimal integer string=w208:string)  [unwired: 1 in]
            n108 = Number To Fractional String(number=w214) -> (F-format string=w206:string)  [unwired: 3 in]
            n109 = case shown="1" w213 {
              tunnel: w214 -> [w220 w222 w231 _]
              frame 0, Default {
                # "controls white light"
                n110 = call-poly <vilib>:"DAQmx Write.vi"("task/channels in"=refnum<k21> "WhiteIntensity1", "data"=w220) -> ()  [unwired: 11 in, 3 out]
              }
              frame 1 {
                n111 = stacked-sequence {
                  tunnel: w222 -> [w223 _ _ _ _]
                  frame #0 {
                    n112 = call-poly <vilib>:"DAQmx Write.vi"("task/channels in"=refnum<k21> "TapStrength1", "data"=w223) -> ()  [unwired: 11 in, 3 out]
                  }
                  frame #1 {
                    n113 = Wait (ms)(milliseconds to wait=u32 500) -> ()  [unwired: 1 out]
                  }
                  frame #2 {
                    n114 = call-poly <vilib>:"DAQmx Write.vi"("task/channels in"=refnum<k21> "TapNow1", "data"=FALSE) -> ()  [unwired: 11 in, 3 out]
                  }
                  frame #3 {
                    n115 = Wait (ms)(milliseconds to wait=u32 10) -> ()  [unwired: 1 out]
                  }
                  frame #4 {
                    n116 = call-poly <vilib>:"DAQmx Write.vi"("task/channels in"=refnum<k21> "TapNow1", "data"=TRUE) -> ()  [unwired: 11 in, 3 out]
                  }
                }
              }
              frame 2 {
                n117 = stacked-sequence {
                  tunnel: w231 -> [_ w234 _]
                  frame #0 {
                    n118 = call-poly <vilib>:"DAQmx Write.vi"("task/channels in"=refnum<k21> "WhiteIntensity1", "data"=5.0) -> ()  [unwired: 11 in, 3 out]
                  }
                  frame #1 {
                    n119 = Wait (ms)(milliseconds to wait=w234) -> ()  [unwired: 1 out]
                  }
                  frame #2 {
                    n120 = call-poly <vilib>:"DAQmx Write.vi"("task/channels in"=refnum<k21> "WhiteIntensity1", "data"=0.0) -> ()  [unwired: 11 in, 3 out]
                  }
                }
              }
              frame 3 {
              }
            }
            n121 = Concatenate Strings(w210, "\r", w208, "\r", w206, "\r") -> (w212:string)
            n122 = local read "event log"() -> (w216:refnum<file>)
            n123 = Write to Text File(file (use dialog)=w216, text=w212) -> (refnum out=w215:refnum<file>)  [unwired: 2 in, 2 out]
            n124 = local write "event log"(w215) -> ()
          }
          frame True {
          }
        }
        n125 = local read "stop"() -> (w204:bool)
      }
      n126 = call "IMAQ Create"("Image Name"="main1") -> ("New Image"=w160:T2)  [unwired: 4 in, 1 out]
      n127 = while {
        tunnel: w145 -> [w268]
        tunnel: w160 -> [w280]
        tunnel: w147 -> [w270]
        tunnel: w143 -> [w266]
        tunnel: w142 -> [w262]
        tunnel: w146 -> [w264]
        tunnel: w144 -> [w263]
        tunnel: w141 -> [w259]
        tunnel: w140 -> [w258]
        i -> [w254]
        stop <- w279 stop-if-true
        n128 = Get Queue Status(queue=w258) -> (# elements in queue=w256:i32)  [unwired: 2 in, 7 out]
        n129 = Get Queue Status(queue=w259) -> (# elements in queue=w257:i32)  [unwired: 2 in, 7 out]
        n130 = case shown="False" "Camera" {
          tunnel: w270 -> [_ w286]
          tunnel: [w283 w286] -> w269
          tunnel: [w282 w285] -> w267
          tunnel: w268 -> [_ w285]
          tunnel: w266 -> [_ w284]
          tunnel: [w281 w284] -> w265
          tunnel: w264 -> [w283 _]
          tunnel: w263 -> [w282 _]
          tunnel: w262 -> [w281 _]
          frame False {
          }
          frame True {
          }
        }
        n131 = Max & Min(x=w257, y=w256) -> (max(x,y)=→"Buffers":i32)  [unwired: 1 out]
        n132 = Quotient & Remainder(x=w254, y=90) -> (x-y*floor(x/y)=w272:i32)  [unwired: 1 out]
        n133 = case shown="1" "Ring" {
          tunnel: w267 -> [w291 _]
          tunnel: [w291 w292] -> w275
          tunnel: w269 -> [_ w292]
          frame 0, Default {
          }
          frame 1 {
          }
        }
        n134 = Equal To 0?(x=w272) -> (x = 0?=w271:bool)
        n135 = case shown="True" w271 {
          tunnel: w265 -> [_ w290]
          frame False {
          }
          frame True {
            n136 = Dequeue Element(queue=w290, timeout in ms (-1)=100) -> (element=w288:u32[][])  [unwired: 1 in, 3 out]
            n137 = Transpose 2D Array(2D array=w288) -> (transposed array=→"Intensity Graph":u32[][])
          }
        }
        n138 = Dequeue Element(queue=w275, timeout in ms (-1)=100) -> (element=w276:u8[][], error out=w278:errorcluster)  [unwired: 1 in, 2 out]
        n139 = call "IMAQ ArrayToImage"("error in (no error)"=w278, "Image Pixels (U8)"=w276, "Image"=w280) -> ("Image Out"=→"Image":T2)  [unwired: 7 in, 1 out]
        n140 = local read "stop"() -> (w279:bool)
      }
      n141 = local read "doQueue2"() -> (w138:refnum<queue>)
      n142 = while {
        stop <- w238 stop-if-true
        n143 = event shown="[3] Key Up" {
          selector: _ -> [_ _ _ _]
          dyn-events: _ -> [_ _ _ _]
          timeout: 100 -> [_ _ _ _]
          event Timeout {
            n144 = event-data() -> ()  [unwired: 1 in, 2 out]
          }
          event "Ring": Value Change {
            n145 = event-data() -> ("NewVal"=w239:u16)  [unwired: 1 in, 4 out]
            n146 = case shown="2" w239 {
              frame 0, Default {
                w242 = u32 0 items=["Grayscale", "Binary", "Gradient", "Rainbow", "Temperature", "User Defined"] ("Palette:Palette Type")
                n147 = property on="Image" class="ImageControl"("Palette Type"=w242) -> ()  [unwired: 2 in, 2 out]
                n148 = property on="Intensity Graph" class="IntGraph (strict)"("Visible"=FALSE) -> ()  [unwired: 2 in, 2 out]
                n149 = property on="Image" class="ImageControl"("Visible"=TRUE) -> ()  [unwired: 2 in, 2 out]
              }
              frame 1 {
                w245 = u32 1 items=["Grayscale", "Binary", "Gradient", "Rainbow", "Temperature", "User Defined"] ("Palette:Palette Type")
                n150 = property on="Image" class="ImageControl"("Palette Type"=w245) -> ()  [unwired: 2 in, 2 out]
                n151 = property on="Intensity Graph" class="IntGraph (strict)"("Visible"=FALSE) -> ()  [unwired: 2 in, 2 out]
                n152 = property on="Image" class="ImageControl"("Visible"=TRUE) -> ()  [unwired: 2 in, 2 out]
              }
              frame 2 {
                n153 = property on="Intensity Graph" class="IntGraph (strict)"("Visible"=TRUE) -> ()  [unwired: 2 in, 2 out]
                n154 = property on="Image" class="ImageControl"("Visible"=FALSE) -> ()  [unwired: 2 in, 2 out]
              }
            }
          }
          event Key Down {
            n155 = event-data() -> ("Char"=w250:i16)  [unwired: 1 in, 4 out]
            n156 = Equal?(x=w250, y=i16 32) -> (x = y?=w248:bool)
            n157 = case shown="True" w248 {
              frame False {
              }
              frame True {
                n158 = local read "Camera"() -> (w251:bool)
                n159 = case shown="True" w251 {
                  frame False {
                    n160 = local read "ROIs 2"() -> (w252:T1)
                    n161 = property on="Image" class="ImageControl"("ROI"=w252) -> ()  [unwired: 2 in, 2 out]
                  }
                  frame True {
                    n162 = local read "ROIs"() -> (w253:T1)
                    n163 = property on="Image" class="ImageControl"("ROI"=w253) -> ()  [unwired: 2 in, 2 out]
                  }
                }
              }
            }
          }
          event Key Up {
            n164 = event-data() -> ()  [unwired: 1 in, 7 out]
            n165 = invoke on="Image" class="ImageControl" method="Clear ROI"() -> ()  [unwired: 3 in, 3 out]
          }
        }
        n166 = local read "stop"() -> (w238:bool)
      }
      n167 = while {
        tunnel: w138 -> [w166]
        stop <- w167 stop-if-true
        n168 = Dequeue Element(queue=w166, timeout in ms (-1)=100) -> (element=w164:dbl[], timed out?=w163:bool)  [unwired: 1 in, 2 out]
        n169 = case shown="False" w163 {
          tunnel: w164 -> [w182 _]
          frame False {
            n170 = local read "frame#2"() -> (w179:i32)
            n171 = Index Array(array=w182, index #1=0 ("index"), index #2=1 ("index")) -> (element #1=w178:dbl, element #2=w177:dbl)
            n172 = Number To Decimal String(number=w179) -> (decimal integer string=w173:string)  [unwired: 1 in]
            n173 = Number To Decimal String(number=w178) -> (decimal integer string=w171:string)  [unwired: 1 in]
            n174 = Number To Fractional String(number=w177) -> (F-format string=w169:string)  [unwired: 3 in]
            n175 = case shown="1" w178 {
              tunnel: w177 -> [w183 w185 w194]
              frame 0, Default {
                n176 = call-poly <vilib>:"DAQmx Write.vi"("task/channels in"=refnum<k21> "WhiteIntensity2", "data"=w183) -> ()  [unwired: 11 in, 3 out]
              }
              frame 1 {
                n177 = stacked-sequence {
                  tunnel: w185 -> [w186 _ _ _ _]
                  frame #0 {
                    n178 = call-poly <vilib>:"DAQmx Write.vi"("task/channels in"=refnum<k21> "TapStrength2", "data"=w186) -> ()  [unwired: 11 in, 3 out]
                  }
                  frame #1 {
                    n179 = Wait (ms)(milliseconds to wait=u32 500) -> ()  [unwired: 1 out]
                  }
                  frame #2 {
                    n180 = call-poly <vilib>:"DAQmx Write.vi"("task/channels in"=refnum<k21> "TapNow2", "data"=FALSE) -> ()  [unwired: 11 in, 3 out]
                  }
                  frame #3 {
                    n181 = Wait (ms)(milliseconds to wait=u32 10) -> ()  [unwired: 1 out]
                  }
                  frame #4 {
                    n182 = call-poly <vilib>:"DAQmx Write.vi"("task/channels in"=refnum<k21> "TapNow2", "data"=TRUE) -> ()  [unwired: 11 in, 3 out]
                  }
                }
              }
              frame 2 {
                n183 = stacked-sequence {
                  tunnel: w194 -> [_ w197 _]
                  frame #0 {
                    n184 = call-poly <vilib>:"DAQmx Write.vi"("task/channels in"=refnum<k21> "WhiteIntensity1", "data"=5.0) -> ()  [unwired: 11 in, 3 out]
                  }
                  frame #1 {
                    n185 = Wait (ms)(milliseconds to wait=w197) -> ()  [unwired: 1 out]
                  }
                  frame #2 {
                    n186 = call-poly <vilib>:"DAQmx Write.vi"("task/channels in"=refnum<k21> "WhiteIntensity1", "data"=0.0) -> ()  [unwired: 11 in, 3 out]
                  }
                }
              }
            }
            n187 = local read "event log 2"() -> (w175:refnum<file>)
            n188 = Concatenate Strings(w173, "\r", w171, "\r", w169, "\r") -> (w174:string)
            n189 = Write to Text File(file (use dialog)=w175, text=w174) -> (refnum out=w176:refnum<file>)  [unwired: 2 in, 2 out]
            n190 = local write "event log 2"(w176) -> ()
          }
          frame True {
          }
        }
        n191 = local read "stop"() -> (w167:bool)
      }
    }
  }
